vi "Aux1 IO.vi"() -> ()   [LabVIEW 2020]
uses:
  <vilib>/Platform/TimedLoop/XDataNode/timing_clust.ctl
  <vilib>/Platform/TimedLoop/XDataNode/nitl_modes.ctl
  <vilib>/Platform/TimedLoop/XDataNode/wakeup.ctl
  <vilib>/rvi/Emulation/niFpgaGetClockAttributes.vi
  <vilib>/rvi/Emulation/niFpgaSctlEmulationGetInTimedLoop.vi
  <vilib>/rvi/Emulation/niFpgaEmulationReportErrorSimple.vi
  <vilib>/rvi/eio/common/nirviEmuTemplateMethod_errors.vi
  <vilib>/rvi/Emulation/niFpgaProcessEmulError.vi
  <vilib>/rvi/Emulation/niFpgaCriticalErrorInLSC.vi
  <vilib>/eio/EIONode/EIONode.xnode
  <vilib>/platform/TimedLoop/XDataNode/XDataNode.xnode
  <vilib>/Platform/TimedLoop/XDataNode/XDNodeRunTimeDep.lvlib
  Front Panel Globals.vi
panel:
  out "Accelerometer Data":sgl[](array[numeric])
  out "Current Data":sgl[](array[numeric])
  out "Current Looprate":sgl
  out "Accelerometer Looprate":sgl
  out "Voltage Data":sgl[](array[numeric])
  out "Voltage Looprate":sgl
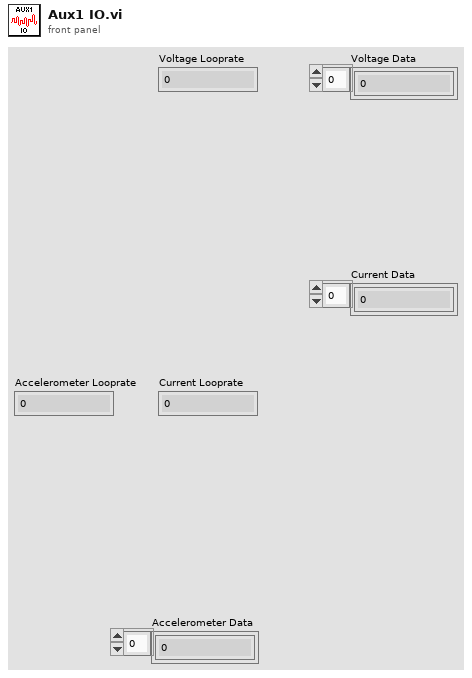
[diagram p1: front panel]
types:
  T1 = typedef "XDNodeRunTimeDep.lvlib/timing_clust.ctl" = cluster{"Expected End [f-1]":u64, "Actual End [f-1]":u64, "Finished Late? [f-1]":bool, "Expected End [i-1]":u64, "Actual End [i-1]":u64, "Finished Late? [i-1]":bool, "Expected Start [i]":u64, "Actual Start [i]":u64, "Expected Start [f]":u64, "Actual Start [f]":u64, "Source Name":string, "Structure Name":string, "Period":i64, "Deadline":i64, "Offset":i64, "Start":i64, "Priority":i32, "Timeout":i32, "Mode":T2, "Wakeup Reason":T3, "Error":errorcluster, "Source Type":string, "Secondary Source Type":string, "Global End Time":u64, "Global Start Time":u64, "Frame Duration":u64, "Iteration Duration":u64, "Assigned CPU":i32, "I/O Scan Engine Mode":u32}
  T2 = typedef "XDNodeRunTimeDep.lvlib/nitl_modes.ctl" = enum32{"No Change", "Process missed periods, maintain original phase", "Discard missed periods, maintain original phase", "Process missed periods, ignore original phase", "Discard missed periods, ignore original phase"}
  T3 = typedef "XDNodeRunTimeDep.lvlib/wakeup.ctl" = enum32{"Normal", "Aborted", "Asynchronous wakeup", "Timing source error", "Timed loop error", "Timeout"}
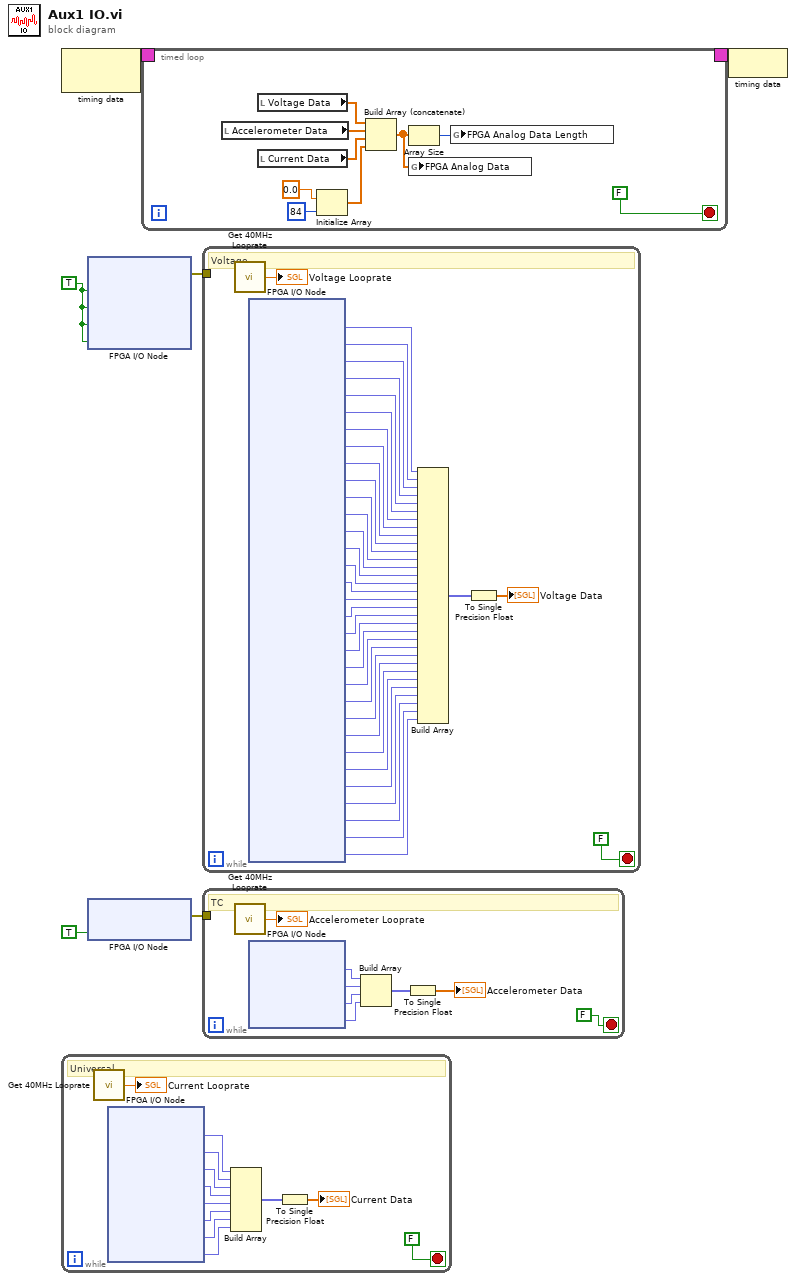
[diagram p0: block diagram]
diagram:
  w4 = TRUE ("Mod1/Start")
  n1 = node-c288() -> (w6:T1)  [unwired: 1 in]
  n2 = while {
    stop <- FALSE stop-if-true
    # "Universal"
    n3 = call "Get 40MHz Looprate.vi"() -> ("Looprate"=→"Current Looprate":sgl)  [unwired: 5 in]
    n4 = xnode "FPGA I/O Node"() -> ("Mod6/AI0"=w16:fxp<+/-,21,-4>, "Mod6/AI1"=w15:fxp<+/-,21,-4>, "Mod6/AI2"=w14:fxp<+/-,21,-4>, "Mod6/AI3"=w13:fxp<+/-,21,-4>, "Mod6/AI4"=w12:fxp<+/-,21,-4>, "Mod6/AI5"=w11:fxp<+/-,21,-4>, "Mod6/AI6"=w10:fxp<+/-,21,-4>, "Mod6/AI7"=w9:fxp<+/-,21,-4>)  [unwired: 8 in, 8 out]
    n5 = Build Array(w16, w15, w14, w13, w12, w11, w10, w9) -> (w7:fxp<+/-,21,-4>[])
    n6 = To Single Precision Float(number=w7) -> (single precision float=→"Current Data":sgl[])
  }
  n7 = xnode "FPGA I/O Node"("Mod1/Start"=w4, "Mod2/Start"=w4, "Mod3/Start"=w4, "Mod4/Start"=w4) -> ("error out"=w3:errorcluster)  [unwired: 5 in, 4 out]
  n8 = xnode "FPGA I/O Node"("Mod5/Start"=TRUE) -> ("error out"=w1:errorcluster)  [unwired: 2 in, 1 out]
  n9 = timed-loop {
    timing: w6 -> [_]
    timing-out: [_] -> w5
    stop <- FALSE stop-if-true
    n10 = local read "Accelerometer Data"() -> (w20:sgl[])
    n11 = local read "Voltage Data"() -> (w21:sgl[])
    n12 = local read "Current Data"() -> (w19:sgl[])
    n13 = Initialize Array(sgl 0.0 ("element"), 84 ("dimension size")) -> (w23:sgl[])
    n14 = Build Array (concatenate)(w21, w20, w19, w23) -> (w26:sgl[])
    n15 = Array Size(array=w26) -> (size(s)=w22:i32)
    n16 = global write "Front Panel Globals.vi" "FPGA Analog Data"(w26) -> ()
    n17 = global write "Front Panel Globals.vi" "FPGA Analog Data Length"(w22) -> ()
  }
  n18 = while {
    tunnel: w3 -> [_]
    stop <- FALSE stop-if-true
    # "Voltage"
    n19 = call "Get 40MHz Looprate.vi"() -> ("Looprate"=→"Voltage Looprate":sgl)  [unwired: 5 in]
    n20 = xnode "FPGA I/O Node"() -> ("Mod1/AI0"=w63:fxp<+/-,24,5>, "Mod1/AI1"=w62:fxp<+/-,24,5>, "Mod1/AI2"=w61:fxp<+/-,24,5>, "Mod1/AI3"=w60:fxp<+/-,24,5>, "Mod1/AI4"=w59:fxp<+/-,24,5>, "Mod1/AI5"=w58:fxp<+/-,24,5>, "Mod1/AI6"=w57:fxp<+/-,24,5>, "Mod1/AI7"=w56:fxp<+/-,24,5>, "Mod2/AI0"=w55:fxp<+/-,24,5>, "Mod2/AI1"=w54:fxp<+/-,24,5>, "Mod2/AI2"=w53:fxp<+/-,24,5>, "Mod2/AI3"=w52:fxp<+/-,24,5>, "Mod2/AI4"=w51:fxp<+/-,24,5>, "Mod2/AI5"=w50:fxp<+/-,24,5>, "Mod2/AI6"=w49:fxp<+/-,24,5>, "Mod2/AI7"=w48:fxp<+/-,24,5>, "Mod3/AI0"=w47:fxp<+/-,24,5>, "Mod3/AI1"=w46:fxp<+/-,24,5>, "Mod3/AI2"=w45:fxp<+/-,24,5>, "Mod3/AI3"=w44:fxp<+/-,24,5>, "Mod3/AI4"=w43:fxp<+/-,24,5>, "Mod3/AI5"=w42:fxp<+/-,24,5>, "Mod3/AI6"=w41:fxp<+/-,24,5>, "Mod3/AI7"=w40:fxp<+/-,24,5>, "Mod4/AI0"=w39:fxp<+/-,24,5>, "Mod4/AI1"=w38:fxp<+/-,24,5>, "Mod4/AI2"=w37:fxp<+/-,24,5>, "Mod4/AI3"=w36:fxp<+/-,24,5>, "Mod4/AI4"=w35:fxp<+/-,24,5>, "Mod4/AI5"=w34:fxp<+/-,24,5>, "Mod4/AI6"=w33:fxp<+/-,24,5>, "Mod4/AI7"=w32:fxp<+/-,24,5>)  [unwired: 32 in, 32 out]
    n21 = Build Array(w63, w62, w61, w60, w59, w58, w57, w56, w55, w54, w53, w52, w51, w50, w49, w48, w47, w46, w45, w44, w43, w42, w41, w40, w39, w38, w37, w36, w35, w34, w33, w32) -> (w30:fxp<+/-,24,5>[])
    n22 = To Single Precision Float(number=w30) -> (single precision float=→"Voltage Data":sgl[])
  }
  n23 = while {
    tunnel: w1 -> [_]
    stop <- FALSE stop-if-true
    # "TC"
    n24 = call "Get 40MHz Looprate.vi"() -> ("Looprate"=→"Accelerometer Looprate":sgl)  [unwired: 5 in]
    n25 = xnode "FPGA I/O Node"() -> ("Mod5/AI0"=w71:fxp<+/-,24,4>, "Mod5/AI1"=w70:fxp<+/-,24,4>, "Mod5/AI2"=w69:fxp<+/-,24,4>, "Mod5/AI3"=w68:fxp<+/-,24,4>)  [unwired: 4 in, 4 out]
    n26 = Build Array(w71, w70, w69, w68) -> (w66:fxp<+/-,24,4>[])
    n27 = To Single Precision Float(number=w66) -> (single precision float=→"Accelerometer Data":sgl[])
  }
  n28 = node-c288(w5) -> ()
